vi "Create Special Real Matrix.vi"(0 "matrix type":i32(ring) items=["Identity", "Diagonal", "Toeplitz", "Vandermonde", "Companion", "Hankel", "Hadamard", "Wilkinson", "Hilbert", "Inverse Hilbert", "Rosser", "Pascal"], 1 "matrix size":i32, 3 "Input Vector1":dbl[](array[numeric]) format="%.2f", 4 "Input Vector2":dbl[](array[numeric]) format="%.2f") -> (5 "Special Matrix":T1, 6 "error":i32)   [LabVIEW 2017, in "NI_AALPro.lvlib"]
doc: "Generates a special matrix based on <B>matrix type</B>. The data types you wire to the <B>Input Vector2</B> and <B>Input Vector1</B> inputs determine the polymorphic instance to use."
uses:
  NI_AALPro.lvlib
  RealMatrix.ctl
  NI_Matrix.lvlib
  <resource>/lvanlys.dll
panel:
  # "Create Special Matrix"
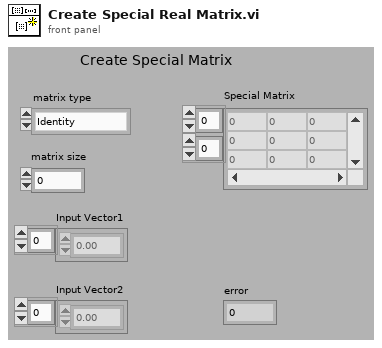
[diagram p1: front panel]
types:
  T1 = typedef "NI_Matrix.lvlib/RealMatrix.ctl" = dbl[][]
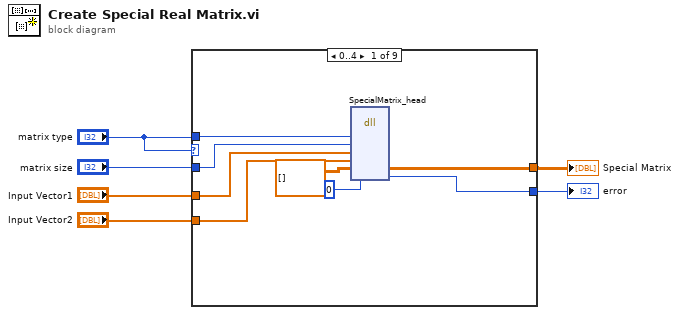
[diagram p0: block diagram]
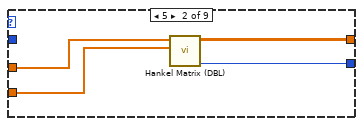
[diagram p2: hidden frame]
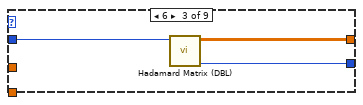
[diagram p3: hidden frame]
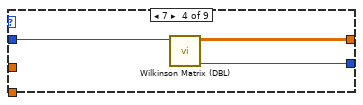
[diagram p4: hidden frame]
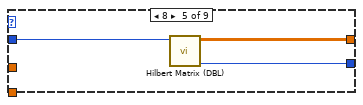
[diagram p5: hidden frame]
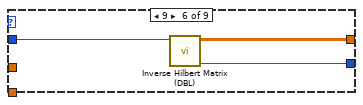
[diagram p6: hidden frame]
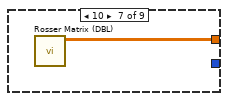
[diagram p7: hidden frame]
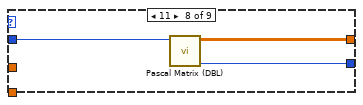
[diagram p8: hidden frame]
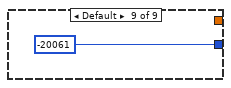
[diagram p9: hidden frame]
diagram:
  n1 = case shown="0..4" "matrix type" {
    tunnel: "matrix type" -> [w12 _ _ _ _ _ _ _ _]
    tunnel: "matrix size" -> [w11 _ w20 w22 w26 w29 _ w33 _]
    tunnel: "Input Vector1" -> [w10 w17 _ _ _ _ _ _ _]
    tunnel: "Input Vector2" -> [w9 w16 _ _ _ _ _ _ _]
    tunnel: [w8 w15 w19 w24 w25 w28 w31 w32 _] -> w2
    tunnel: [w7 w18 w21 w23 w27 w30 _ w34 -20061] -> w1
    frame 0..4 {
      n2 = dll-call lib="C:/Program Files (x86)/National Instruments/LabVIEW 2017/resource/lvanlys.*" fn="SpecialMatrix_head"("matrix type"=w12, "matrix size"=w11, "Input Vector1"=w10, "Input Vector2"=w9, "Special Matrix"=T1 [], 0) -> ("Special Matrix"=w8:T1, w7:i32)  [unwired: 8 in, 2 out]
    }
    frame 5 {
      n3 = call "Hankel Matrix (DBL).vi"("Input Vector2"=w16, "Input Vector1"=w17) -> ("error"=w18:i32, "Hankel Matrix"=w15:T1)  [unwired: 8 in]
    }
    frame 6 {
      n4 = call "Hadamard Matrix (DBL).vi"("matrix size"=w20) -> ("error"=w21:i32, "Hadamard Matrix"=w19:T1)  [unwired: 9 in]
    }
    frame 7 {
      n5 = call "Wilkinson Matrix (DBL).vi"("matrix size"=w22) -> ("error"=w23:i32, "Wilkinson Matrix"=w24:T1)  [unwired: 9 in]
    }
    frame 8 {
      n6 = call "Hilbert Matrix (DBL).vi"("matrix size"=w26) -> ("error"=w27:i32, "Hilbert Matrix"=w25:T1)  [unwired: 9 in]
    }
    frame 9 {
      n7 = call "Inverse Hilbert Matrix (DBL).vi"("matrix size"=w29) -> ("error"=w30:i32, "Inverse Hilbert Matrix"=w28:T1)  [unwired: 9 in]
    }
    frame 10 {
      n8 = call "Rosser Matrix (DBL).vi"() -> ("Rosser Matrix"=w31:T1)  [unwired: 11 in]
    }
    frame 11 {
      n9 = call "Pascal Matrix (DBL).vi"("matrix size"=w33) -> ("error"=w34:i32, "Pascal Matrix"=w32:T1)  [unwired: 9 in]
    }
    frame Default {
    }
  }
  "Special Matrix" <- w2
  "error" <- w1
